vi "Add Information Channels.vi"(8 "error in (no error)":errorcluster, 11 "Node Ptr":u64) -> (0 "error out":errorcluster, 3 "Parent Ref out":T1 format="%.0x")   [LabVIEW 2015, in "Protection and Counter Addon System Explorer.lvlib"]
uses:
  Protection and Counter Addon System Explorer.lvlib
  <vilib>/NI Veristand/Custom Device API/Custom Device Item Ref.ctl
  <vilib>/NI Veristand/Custom Device API/Custom Device Channel.ctl
  <vilib>/NI Veristand/Custom Device API/Custom Device Channel Type.ctl
  Shared/SubVIs/GUID Lookup.vi
  <vilib>/NI VeriStand/Custom Device API/Custom Device API.lvlib
  <vilib>/NI/NI VeriStand Advanced SysDef API/SysDef API/Advanced System Definition.lvlib
  Shared/Protection and Counter Addon Shared.lvlib
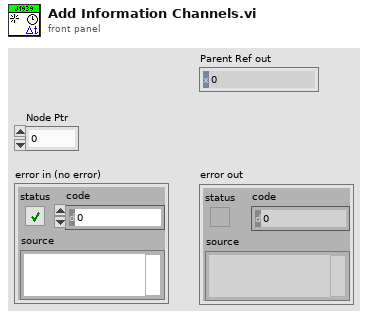
[diagram p1: front panel]
types:
  T1 = typedef "Custom Device API.lvlib/Custom Device Item Ref.ctl" = u64
  T2 = typedef "Custom Device API.lvlib/Custom Device Channel.ctl" = cluster{"Type":T3, "Units":string, "Default Value":dbl, "Faultable":bool, "Scalable":bool}
  T3 = typedef "Custom Device API.lvlib/Custom Device Channel Type.ctl" = enum16{"Input", "Output"}
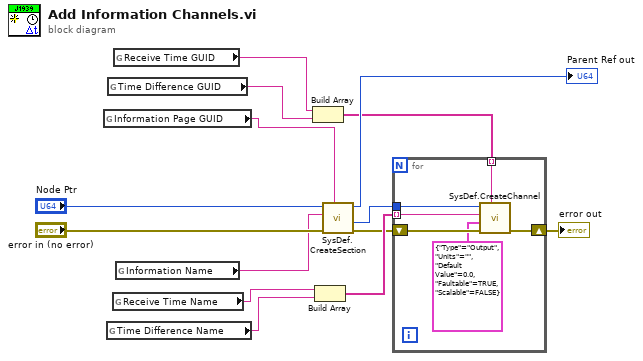
[diagram p0: block diagram]
diagram:
  n1 = global read "GUID Lookup.vi" "Information Page GUID"() -> (w4:string)
  n2 = global read "GUID Lookup.vi" "Time Difference Name"() -> (w1:string)
  n3 = global read "GUID Lookup.vi" "Time Difference GUID"() -> (w5:string)
  n4 = global read "GUID Lookup.vi" "Receive Time Name"() -> (w2:string)
  n5 = global read "GUID Lookup.vi" "Receive Time GUID"() -> (w6:string)
  n6 = global read "GUID Lookup.vi" "Information Name"() -> (w3:string)
  n7 = Build Array(w6, w5) -> (w13:string[])
  n8 = Build Array(w2, w1) -> (w12:string[])
  n9 = call <vilib>:"SysDef.CreateSection.vi"("GUID"=w4, "error in (no error)"="error in (no error)", "Name"=w3, "nodeID"="Node Ptr") -> ("error out"=w8:errorcluster, "New NodeID"=w9:u64, "nodeID out"=→"Parent Ref out":u64)  [unwired: 4 in, 1 out]
  n10 = for {
    tunnel: w9 -> [w19]
    shift-right: [w18] -> w11
    shift-left: w8 -> [w20]
    tunnel: w13 -> [w16] mode=indexing
    tunnel: w12 -> [w15] mode=indexing
    n11 = call <vilib>:"SysDef.CreateChannel.vi"("GUID"=w16, "error in (no error)"=w20, "Channel"=T2 {"Type"=enum."Output", "Units"="", "Default Value"=0.0, "Faultable"=TRUE, "Scalable"=FALSE}, "Name"=w15, "nodeID"=w19) -> ("error out"=w18:errorcluster)  [unwired: 3 in, 3 out]
  }
  "error out" <- w11
